vi "MFC log.vi"(9 "SetPoint (64000=FullScale)":i32=32000 min=0 max=64000 step=1, 10 "UnitID":string="A", 11 "VISA resource name":refnum<visa-resource-name>="COM1") -> (0 "error out":errorcluster={"status"=FALSE, "code"=0, "source"="VISA Read in ReadSerialBuffer.vi->AlicatSetPoint.vi->AlicatWrite8V2.vi"}, 1 "AlicatResponse":string="A +013.53 +023.20 +0000.0 +0000.0 0250.0     Air\r")   [LabVIEW 2011]
uses:
  <vilib>/Instr/_visa.llb/VISA Configure Serial Port (Instr).vi
  <vilib>/Utility/file.llb/Write To Spreadsheet File (DBL).vi
panel:
  out "Array 2":i32[](array[numeric])
  in  "File Name":string
  out "Waveform Graph":dbl[](graph)
  out "Array":dbl[][](array[numeric])
  # "Put this first"
  # "0= 0%\n64000 = 100%"
  # "Read this response from the change the setpoint write.\nClears the Serial in buffer"
  # "Code 1073676294 is\nokay since we are only\nreading one byte till we\nget to the end of message\nbyte."
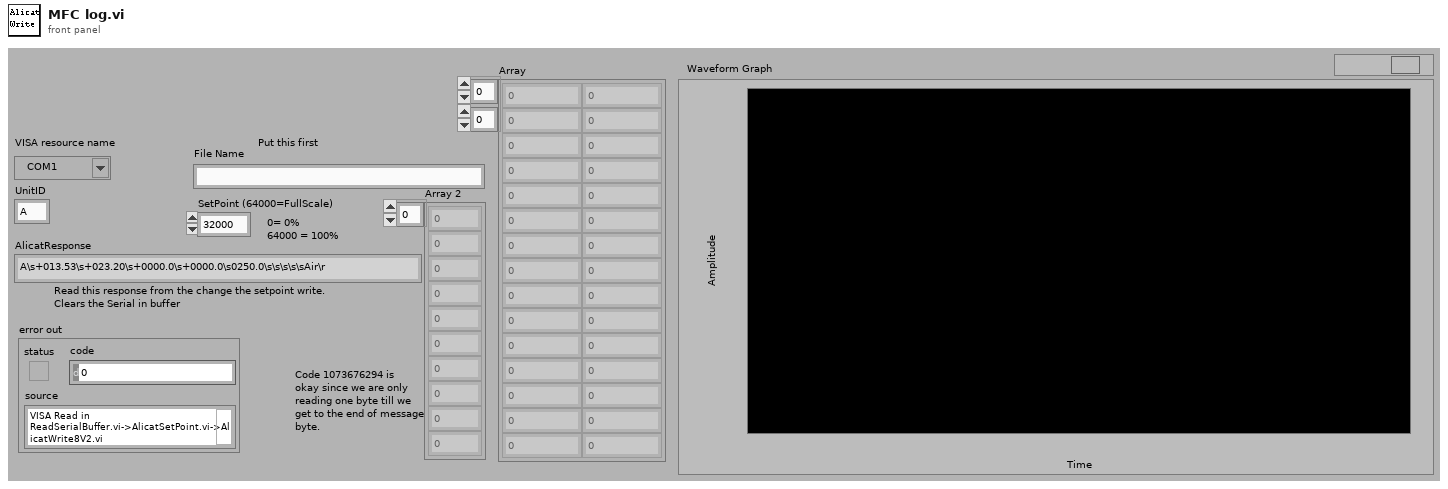
[diagram p1: front panel]
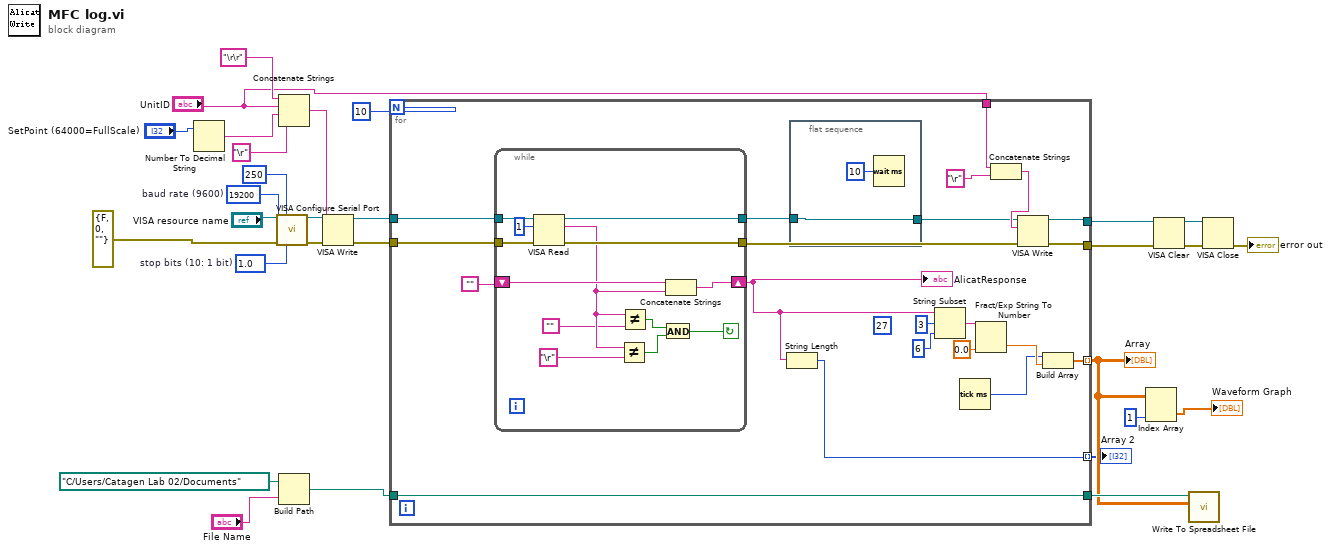
[diagram p0: block diagram]
diagram:
  w27 = u16 10 items=["1.0"=10, "1.5"=15, "2.0"=20]  # stop bits (10: 1 bit)
  w28 = u32 19200  # baud rate (9600)
  n1 = Number To Decimal String(number="SetPoint (64000=FullScale)") -> (decimal integer string=w12:string)  [unwired: 1 in]
  n2 = call-poly "VISA Configure Serial Port"("VISA resource name"="VISA resource name", "timeout (10sec)"=u32 250, "baud rate (9600)"=w28, "error in (no error)"=errorcluster {"status"=FALSE, "code"=0, "source"=""}, "stop bits (10: 1 bit)"=w27) -> ("VISA resource name out"=w24:refnum<visa-resource-name>, "error out"=w23:errorcluster)  [unwired: 9 in]
  n3 = Concatenate Strings("\r\r" ("string"), "UnitID", w12, "\r" ("string")) -> (w15:string)
  n4 = Build Path(base path=path "C:/Users/Catagen Lab 02/Documents", name or relative path="File Name") -> (appended path=w3:path)
  n5 = VISA Write(VISA resource name=w24, write buffer=w15, error in (no error)=w23) -> (VISA resource name out=w17:refnum<visa-resource-name>, error out=w16:errorcluster)  [unwired: 1 out]
  n6 = for {
    N: 10 -> [_]
    tunnel: [w38] -> w22
    tunnel: [w39] -> w21
    tunnel: w17 -> [w40]
    tunnel: w16 -> [w41]
    tunnel: [w45] -> w2 mode=indexing
    tunnel: "UnitID" -> [w35]
    tunnel: [w34] -> w8
    tunnel: w3 -> [w34]
    tunnel: [w30] -> w1 mode=indexing
    (unwired) 27 ("length (rest)")
    n7 = while {
      tunnel: [w64] -> w37
      tunnel: [w63] -> w32
      shift-right: [w61] -> w31
      shift-left: "" -> [w60]
      tunnel: w40 -> [w54]
      tunnel: w41 -> [w53]
      stop <- w56 continue-if-true
      n8 = VISA Read(VISA resource name=w54, byte count=u32 1 ("byte count (0)"), error in (no error)=w53) -> (VISA resource name out=w63:refnum<visa-resource-name>, read buffer=w59:string, error out=w64:errorcluster)  [unwired: 1 out]
      n9 = Not Equal?(x=w59, y="\r") -> (x != y?=w57:bool)
      n10 = Not Equal?(x=w59, y="") -> (x != y?=w58:bool)
      n11 = And(x=w58, y=w57) -> (x .and. y?=w56:bool)
      n12 = Concatenate Strings(w60, w59) -> (w61:string)
    }
    "AlicatResponse" <- w31
    n13 = String Length(string=w31) -> (length=w30:i32)
    n14 = flat-sequence {
      tunnel: [w52] -> w33
      tunnel: w32 -> [w52]
      frame #0 {
        n15 = Wait (ms)(milliseconds to wait=u32 10) -> ()  [unwired: 1 out]
      }
    }
    n16 = String Subset(string=w31, offset (0)=3 ("length (rest)"), length (rest)=6 ("offset (0)")) -> (substring=w47:string)
    n17 = Tick Count (ms)() -> (millisecond timer value=w36:u32)
    n18 = Fract/Exp String To Number(string=w47, default (0 dbl)=0.0) -> (number=w44:dbl)  [unwired: 2 in, 1 out]
    n19 = Concatenate Strings(w35, "\r" ("string")) -> (w42:string)
    n20 = VISA Write(VISA resource name=w33, write buffer=w42, error in (no error)=w37) -> (VISA resource name out=w38:refnum<visa-resource-name>, error out=w39:errorcluster)  [unwired: 1 out]
    n21 = Build Array(w36, w44) -> (w45:dbl[])
  }
  "Array" <- w2
  "Array 2" <- w1
  n22 = Index Array(array=w2, index (col)=1 ("disabled index (col)")) -> (element=→"Waveform Graph":dbl[])  [unwired: 1 in]
  n23 = VISA Clear(VISA resource name=w22, error in (no error)=w21) -> (VISA resource name out=w19:refnum<visa-resource-name>, error out=w18:errorcluster)
  n24 = call-poly <vilib>:"Write To Spreadsheet File.vi"("2D data"=w2, "file path (dialog if empty)"=w8) -> ()  [unwired: 6 in, 1 out]
  n25 = VISA Close(VISA resource name=w19, error in (no error)=w18) -> (error out=→"error out":errorcluster)
